vi "ZK流程写入.vi"(7 "是否启用通讯通知":bool, 8 "error in (no error)":errorcluster, 10 "流程":T1 {"进样流程"."进样流程-进样"."步骤二："."功能" items=["加标", "进样", "排液", "搅拌", "定量", "延时"]; "进样流程"."进样流程-进样"."步骤一："."功能" items=["加标", "进样", "排液", "搅拌", "定量", "延时"]; "进样流程"."进样流程-进样"."步骤四："."功能" items=["加标", "进样", "排液", "搅拌", "定量", "延时"]; "进样流程"."进样流程-进样"."步骤三："."功能" items=["加标", "进样", "排液", "搅拌", "定量", "延时"]; "进样流程"."进样流程-进样"."步骤六："."功能" items=["加标", "进样", "排液", "搅拌", "定量", "延时"]; "进样流程"."进样流程-进样"."步骤五："."功能" items=["加标", "进样", "排液", "搅拌", "定量", "延时"]; "进样流程"."进样流程-进样"."步骤八："."功能" items=["加标", "进样", "排液", "搅拌", "定量", "延时"]; "进样流程"."进样流程-进样"."步骤七："."功能" items=["加标", "进样", "排液", "搅拌", "定量", "延时"]; "进样流程"."进样流程-进样"."步骤十："."功能" items=["加标", "进样", "排液", "搅拌", "定量", "延时"]; "进样流程"."进样流程-进样"."步骤九："."功能" items=["加标", "进样", "排液", "搅拌", "定量", "延时"]; "进样流程"."进样流程-润洗"."步骤二："."功能" items=["加标", "进样", "排液", "搅拌", "定量", "延时"]; "进样流程"."进样流程-润洗"."步骤一："."功能" items=["加标", "进样", "排液", "搅拌", "定量", "延时"]; "进样流程"."进样流程-润洗"."步骤四："."功能" items=["加标", "进样", "排液", "搅拌", "定量", "延时"]; "进样流程"."进样流程-润洗"."步骤三："."功能" items=["加标", "进样", "排液", "搅拌", "定量", "延时"]; "进样流程"."进样流程-润洗"."步骤六："."功能" items=["加标", "进样", "排液", "搅拌", "定量", "延时"]; "进样流程"."进样流程-润洗"."步骤五："."功能" items=["加标", "进样", "排液", "搅拌", "定量", "延时"]; "进样流程"."进样流程-润洗"."步骤八："."功能" items=["加标", "进样", "排液", "搅拌", "定量", "延时"]; "进样流程"."进样流程-润洗"."步骤七："."功能" items=["加标", "进样", "排液", "搅拌", "定量", "延时"]; "进样流程"."进样流程-润洗"."步骤十："."功能" items=["加标", "进样", "排液", "搅拌", "定量", "延时"]; "进样流程"."进样流程-润洗"."步骤九："."功能" items=["加标", "进样", "排液", "搅拌", "定量", "延时"]; "排液流程"."步骤二："."功能" items=["加标", "进样", "排液", "搅拌", "定量", "延时"]; "排液流程"."步骤一："."功能" items=["加标", "进样", "排液", "搅拌", "定量", "延时"]; "排液流程"."步骤四："."功能" items=["加标", "进样", "排液", "搅拌", "定量", "延时"]; "排液流程"."步骤三："."功能" items=["加标", "进样", "排液", "搅拌", "定量", "延时"]; "排液流程"."步骤六："."功能" items=["加标", "进样", "排液", "搅拌", "定量", "延时"]; "排液流程"."步骤五："."功能" items=["加标", "进样", "排液", "搅拌", "定量", "延时"]; "排液流程"."步骤八："."功能" items=["加标", "进样", "排液", "搅拌", "定量", "延时"]; "排液流程"."步骤七："."功能" items=["加标", "进样", "排液", "搅拌", "定量", "延时"]; "排液流程"."步骤十："."功能" items=["加标", "进样", "排液", "搅拌", "定量", "延时"]; "排液流程"."步骤九："."功能" items=["加标", "进样", "排液", "搅拌", "定量", "延时"]; "加标流程"."加标流程-加标"."步骤二："."功能" items=["加标", "进样", "排液", "搅拌", "定量", "延时"]; "加标流程"."加标流程-加标"."步骤一："."功能" items=["加标", "进样", "排液", "搅拌", "定量", "延时"]; "加标流程"."加标流程-加标"."步骤四："."功能" items=["加标", "进样", "排液", "搅拌", "定量", "延时"]; "加标流程"."加标流程-加标"."步骤三："."功能" items=["加标", "进样", "排液", "搅拌", "定量", "延时"]; "加标流程"."加标流程-加标"."步骤六："."功能" items=["加标", "进样", "排液", "搅拌", "定量", "延时"]; "加标流程"."加标流程-加标"."步骤五："."功能" items=["加标", "进样", "排液", "搅拌", "定量", "延时"]; "加标流程"."加标流程-加标"."步骤八："."功能" items=["加标", "进样", "排液", "搅拌", "定量", "延时"]; "加标流程"."加标流程-加标"."步骤七："."功能" items=["加标", "进样", "排液", "搅拌", "定量", "延时"]; "加标流程"."加标流程-加标"."步骤十："."功能" items=["加标", "进样", "排液", "搅拌", "定量", "延时"]; "加标流程"."加标流程-加标"."步骤九："."功能" items=["加标", "进样", "排液", "搅拌", "定量", "延时"]; "加标流程"."加标流程-定量"."步骤二："."功能" items=["加标", "进样", "排液", "搅拌", "定量", "延时"]; "加标流程"."加标流程-定量"."步骤一："."功能" items=["加标", "进样", "排液", "搅拌", "定量", "延时"]; "加标流程"."加标流程-定量"."步骤四："."功能" items=["加标", "进样", "排液", "搅拌", "定量", "延时"]; "加标流程"."加标流程-定量"."步骤三："."功能" items=["加标", "进样", "排液", "搅拌", "定量", "延时"]; "加标流程"."加标流程-定量"."步骤六："."功能" items=["加标", "进样", "排液", "搅拌", "定量", "延时"]; "加标流程"."加标流程-定量"."步骤五："."功能" items=["加标", "进样", "排液", "搅拌", "定量", "延时"]; "加标流程"."加标流程-定量"."步骤八："."功能" items=["加标", "进样", "排液", "搅拌", "定量", "延时"]; "加标流程"."加标流程-定量"."步骤七："."功能" items=["加标", "进样", "排液", "搅拌", "定量", "延时"]; "加标流程"."加标流程-定量"."步骤十："."功能" items=["加标", "进样", "排液", "搅拌", "定量", "延时"]; "加标流程"."加标流程-定量"."步骤九："."功能" items=["加标", "进样", "排液", "搅拌", "定量", "延时"]; "加标流程"."加标流程-进样"."步骤二："."功能" items=["加标", "进样", "排液", "搅拌", "定量", "延时"]; "加标流程"."加标流程-进样"."步骤一："."功能" items=["加标", "进样", "排液", "搅拌", "定量", "延时"]; "加标流程"."加标流程-进样"."步骤四："."功能" items=["加标", "进样", "排液", "搅拌", "定量", "延时"]; "加标流程"."加标流程-进样"."步骤三："."功能" items=["加标", "进样", "排液", "搅拌", "定量", "延时"]; "加标流程"."加标流程-进样"."步骤六："."功能" items=["加标", "进样", "排液", "搅拌", "定量", "延时"]; "加标流程"."加标流程-进样"."步骤五："."功能" items=["加标", "进样", "排液", "搅拌", "定量", "延时"]; "加标流程"."加标流程-进样"."步骤八："."功能" items=["加标", "进样", "排液", "搅拌", "定量", "延时"]; "加标流程"."加标流程-进样"."步骤七："."功能" items=["加标", "进样", "排液", "搅拌", "定量", "延时"]; "加标流程"."加标流程-进样"."步骤十："."功能" items=["加标", "进样", "排液", "搅拌", "定量", "延时"]; "加标流程"."加标流程-进样"."步骤九："."功能" items=["加标", "进样", "排液", "搅拌", "定量", "延时"]; "加标流程"."加标流程-润洗"."步骤二："."功能" items=["加标", "进样", "排液", "搅拌", "定量", "延时"]; "加标流程"."加标流程-润洗"."步骤一："."功能" items=["加标", "进样", "排液", "搅拌", "定量", "延时"]; "加标流程"."加标流程-润洗"."步骤四："."功能" items=["加标", "进样", "排液", "搅拌", "定量", "延时"]; "加标流程"."加标流程-润洗"."步骤三："."功能" items=["加标", "进样", "排液", "搅拌", "定量", "延时"]; "加标流程"."加标流程-润洗"."步骤六："."功能" items=["加标", "进样", "排液", "搅拌", "定量", "延时"]; "加标流程"."加标流程-润洗"."步骤五："."功能" items=["加标", "进样", "排液", "搅拌", "定量", "延时"]; "加标流程"."加标流程-润洗"."步骤八："."功能" items=["加标", "进样", "排液", "搅拌", "定量", "延时"]; "加标流程"."加标流程-润洗"."步骤七："."功能" items=["加标", "进样", "排液", "搅拌", "定量", "延时"]; "加标流程"."加标流程-润洗"."步骤十："."功能" items=["加标", "进样", "排液", "搅拌", "定量", "延时"]; "加标流程"."加标流程-润洗"."步骤九："."功能" items=["加标", "进样", "排液", "搅拌", "定量", "延时"]; "加标润洗流程"."步骤二："."功能" items=["加标", "进样", "排液", "搅拌", "定量", "延时"]; "加标润洗流程"."步骤一："."功能" items=["加标", "进样", "排液", "搅拌", "定量", "延时"]; "加标润洗流程"."步骤四："."功能" items=["加标", "进样", "排液", "搅拌", "定量", "延时"]; "加标润洗流程"."步骤三："."功能" items=["加标", "进样", "排液", "搅拌", "定量", "延时"]; "加标润洗流程"."步骤六："."功能" items=["加标", "进样", "排液", "搅拌", "定量", "延时"]; "加标润洗流程"."步骤五："."功能" items=["加标", "进样", "排液", "搅拌", "定量", "延时"]; "加标润洗流程"."步骤八："."功能" items=["加标", "进样", "排液", "搅拌", "定量", "延时"]; "加标润洗流程"."步骤七："."功能" items=["加标", "进样", "排液", "搅拌", "定量", "延时"]; "加标润洗流程"."步骤十："."功能" items=["加标", "进样", "排液", "搅拌", "定量", "延时"]; "加标润洗流程"."步骤九："."功能" items=["加标", "进样", "排液", "搅拌", "定量", "延时"]; "水样润洗流程"."步骤二："."功能" items=["加标", "进样", "排液", "搅拌", "定量", "延时"]; "水样润洗流程"."步骤一："."功能" items=["加标", "进样", "排液", "搅拌", "定量", "延时"]; "水样润洗流程"."步骤四："."功能" items=["加标", "进样", "排液", "搅拌", "定量", "延时"]; "水样润洗流程"."步骤三："."功能" items=["加标", "进样", "排液", "搅拌", "定量", "延时"]; "水样润洗流程"."步骤六："."功能" items=["加标", "进样", "排液", "搅拌", "定量", "延时"]; "水样润洗流程"."步骤五："."功能" items=["加标", "进样", "排液", "搅拌", "定量", "延时"]; "水样润洗流程"."步骤八："."功能" items=["加标", "进样", "排液", "搅拌", "定量", "延时"]; "水样润洗流程"."步骤七："."功能" items=["加标", "进样", "排液", "搅拌", "定量", "延时"]; "水样润洗流程"."步骤十："."功能" items=["加标", "进样", "排液", "搅拌", "定量", "延时"]; "水样润洗流程"."步骤九："."功能" items=["加标", "进样", "排液", "搅拌", "定量", "延时"]}, 11 "Slave ID":T2) -> (0 "error out":errorcluster)   [LabVIEW 2016, in "质控单元V4.lvlib"]
uses:
  <vilib>/Plasmionique/MB Master/MB_Master/MB_Master.lvclass
  <vilib>/Plasmionique/MB Master/MB Master.lvlib
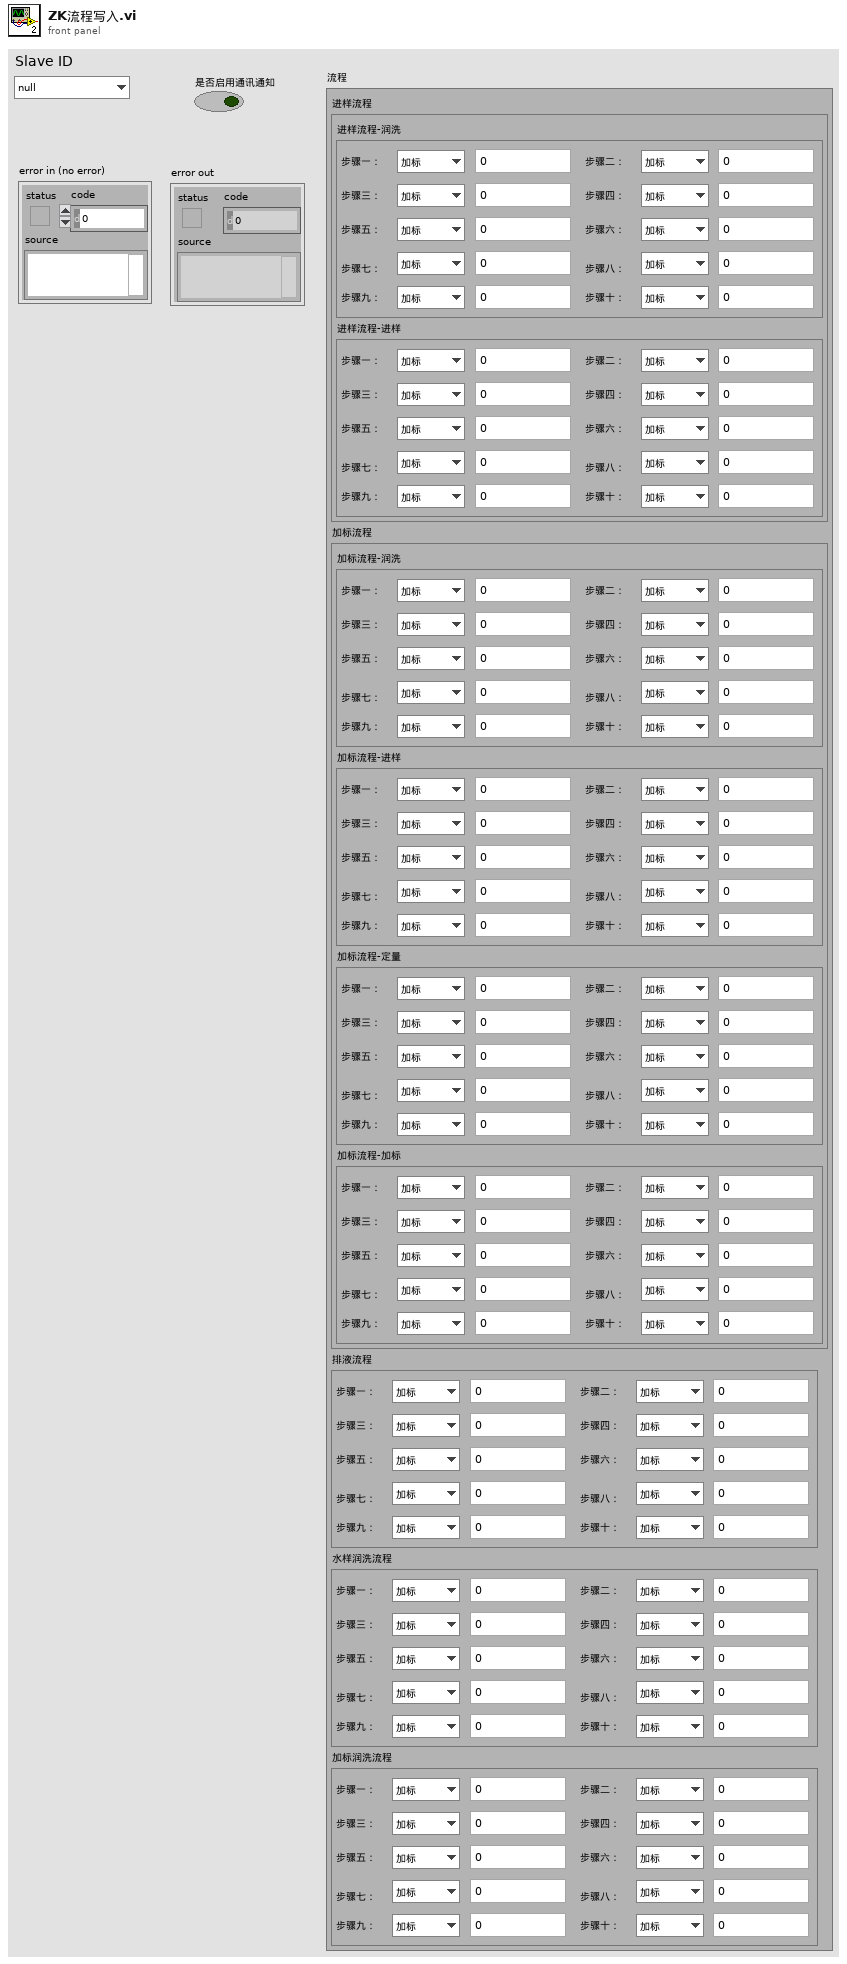
[diagram p1: front panel]
types:
  T1 = cluster{"进样流程":cluster{"进样流程-润洗":cluster{"步骤一：":cluster{"功能":u16, "值":sgl}, "步骤二：":cluster{"功能":u16, "值":sgl}, "步骤三：":cluster{"功能":u16, "值":sgl}, "步骤四：":cluster{"功能":u16, "值":sgl}, "步骤五：":cluster{"功能":u16, "值":sgl}, "步骤六：":cluster{"功能":u16, "值":sgl}, "步骤七：":cluster{"功能":u16, "值":sgl}, "步骤八：":cluster{"功能":u16, "值":sgl}, "步骤九：":cluster{"功能":u16, "值":sgl}, "步骤十：":cluster{"功能":u16, "值":sgl}}, "进样流程-进样":cluster{"步骤一：":cluster{"功能":u16, "值":sgl}, "步骤二：":cluster{"功能":u16, "值":sgl}, "步骤三：":cluster{"功能":u16, "值":sgl}, "步骤四：":cluster{"功能":u16, "值":sgl}, "步骤五：":cluster{"功能":u16, "值":sgl}, "步骤六：":cluster{"功能":u16, "值":sgl}, "步骤七：":cluster{"功能":u16, "值":sgl}, "步骤八：":cluster{"功能":u16, "值":sgl}, "步骤九：":cluster{"功能":u16, "值":sgl}, "步骤十：":cluster{"功能":u16, "值":sgl}}}, "加标流程":cluster{"加标流程-润洗":cluster{"步骤一：":cluster{"功能":u16, "值":sgl}, "步骤二：":cluster{"功能":u16, "值":sgl}, "步骤三：":cluster{"功能":u16, "值":sgl}, "步骤四：":cluster{"功能":u16, "值":sgl}, "步骤五：":cluster{"功能":u16, "值":sgl}, "步骤六：":cluster{"功能":u16, "值":sgl}, "步骤七：":cluster{"功能":u16, "值":sgl}, "步骤八：":cluster{"功能":u16, "值":sgl}, "步骤九：":cluster{"功能":u16, "值":sgl}, "步骤十：":cluster{"功能":u16, "值":sgl}}, "加标流程-进样":cluster{"步骤一：":cluster{"功能":u16, "值":sgl}, "步骤二：":cluster{"功能":u16, "值":sgl}, "步骤三：":cluster{"功能":u16, "值":sgl}, "步骤四：":cluster{"功能":u16, "值":sgl}, "步骤五：":cluster{"功能":u16, "值":sgl}, "步骤六：":cluster{"功能":u16, "值":sgl}, "步骤七：":cluster{"功能":u16, "值":sgl}, "步骤八：":cluster{"功能":u16, "值":sgl}, "步骤九：":cluster{"功能":u16, "值":sgl}, "步骤十：":cluster{"功能":u16, "值":sgl}}, "加标流程-定量":cluster{"步骤一：":cluster{"功能":u16, "值":sgl}, "步骤二：":cluster{"功能":u16, "值":sgl}, "步骤三：":cluster{"功能":u16, "值":sgl}, "步骤四：":cluster{"功能":u16, "值":sgl}, "步骤五：":cluster{"功能":u16, "值":sgl}, "步骤六：":cluster{"功能":u16, "值":sgl}, "步骤七：":cluster{"功能":u16, "值":sgl}, "步骤八：":cluster{"功能":u16, "值":sgl}, "步骤九：":cluster{"功能":u16, "值":sgl}, "步骤十：":cluster{"功能":u16, "值":sgl}}, "加标流程-加标":cluster{"步骤一：":cluster{"功能":u16, "值":sgl}, "步骤二：":cluster{"功能":u16, "值":sgl}, "步骤三：":cluster{"功能":u16, "值":sgl}, "步骤四：":cluster{"功能":u16, "值":sgl}, "步骤五：":cluster{"功能":u16, "值":sgl}, "步骤六：":cluster{"功能":u16, "值":sgl}, "步骤七：":cluster{"功能":u16, "值":sgl}, "步骤八：":cluster{"功能":u16, "值":sgl}, "步骤九：":cluster{"功能":u16, "值":sgl}, "步骤十：":cluster{"功能":u16, "值":sgl}}}, "排液流程":cluster{"步骤一：":cluster{"功能":u16, "值":sgl}, "步骤二：":cluster{"功能":u16, "值":sgl}, "步骤三：":cluster{"功能":u16, "值":sgl}, "步骤四：":cluster{"功能":u16, "值":sgl}, "步骤五：":cluster{"功能":u16, "值":sgl}, "步骤六：":cluster{"功能":u16, "值":sgl}, "步骤七：":cluster{"功能":u16, "值":sgl}, "步骤八：":cluster{"功能":u16, "值":sgl}, "步骤九：":cluster{"功能":u16, "值":sgl}, "步骤十：":cluster{"功能":u16, "值":sgl}}, "水样润洗流程":cluster{"步骤一：":cluster{"功能":u16, "值":sgl}, "步骤二：":cluster{"功能":u16, "值":sgl}, "步骤三：":cluster{"功能":u16, "值":sgl}, "步骤四：":cluster{"功能":u16, "值":sgl}, "步骤五：":cluster{"功能":u16, "值":sgl}, "步骤六：":cluster{"功能":u16, "值":sgl}, "步骤七：":cluster{"功能":u16, "值":sgl}, "步骤八：":cluster{"功能":u16, "值":sgl}, "步骤九：":cluster{"功能":u16, "值":sgl}, "步骤十：":cluster{"功能":u16, "值":sgl}}, "加标润洗流程":cluster{"步骤一：":cluster{"功能":u16, "值":sgl}, "步骤二：":cluster{"功能":u16, "值":sgl}, "步骤三：":cluster{"功能":u16, "值":sgl}, "步骤四：":cluster{"功能":u16, "值":sgl}, "步骤五：":cluster{"功能":u16, "值":sgl}, "步骤六：":cluster{"功能":u16, "值":sgl}, "步骤七：":cluster{"功能":u16, "值":sgl}, "步骤八：":cluster{"功能":u16, "值":sgl}, "步骤九：":cluster{"功能":u16, "值":sgl}, "步骤十：":cluster{"功能":u16, "值":sgl}}}
  T2 = typedef "质控单元V4.lvlib/质控slave id.ctl" = enum16{"null", "氨氮", "总磷", "总氮", "CODMn", "CODCr"}
  T3 = cluster{"步骤一：":cluster{"功能":u16, "值":sgl}, "步骤二：":cluster{"功能":u16, "值":sgl}, "步骤三：":cluster{"功能":u16, "值":sgl}, "步骤四：":cluster{"功能":u16, "值":sgl}, "步骤五：":cluster{"功能":u16, "值":sgl}, "步骤六：":cluster{"功能":u16, "值":sgl}, "步骤七：":cluster{"功能":u16, "值":sgl}, "步骤八：":cluster{"功能":u16, "值":sgl}, "步骤九：":cluster{"功能":u16, "值":sgl}, "步骤十：":cluster{"功能":u16, "值":sgl}}
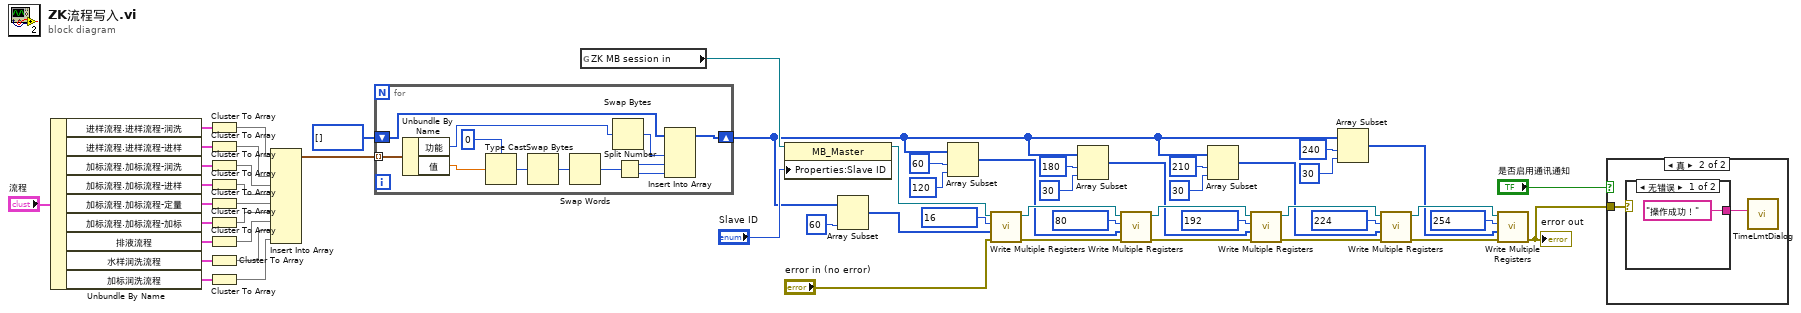
[diagram p0: block diagram]
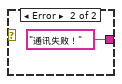
[diagram p3: hidden frame]
diagram:
  n1 = Unbundle By Name("流程") -> ("进样流程.进样流程-润洗"=w48:T3, "进样流程.进样流程-进样"=w46:T3, "加标流程.加标流程-润洗"=w45:T3, "加标流程.加标流程-进样"=w44:T3, "加标流程.加标流程-定量"=w43:T3, "加标流程.加标流程-加标"=w42:T3, "排液流程"=w41:T3, "水样润洗流程"=w40:T3, "加标润洗流程"=w39:T3)
  n2 = Cluster To Array(cluster=w48) -> (array=w38:cluster{"功能":u16, "值":sgl}[])
  n3 = Cluster To Array(cluster=w46) -> (array=w37:cluster{"功能":u16, "值":sgl}[])
  n4 = Cluster To Array(cluster=w45) -> (array=w36:cluster{"功能":u16, "值":sgl}[])
  n5 = Cluster To Array(cluster=w44) -> (array=w35:cluster{"功能":u16, "值":sgl}[])
  n6 = Cluster To Array(cluster=w43) -> (array=w34:cluster{"功能":u16, "值":sgl}[])
  n7 = Cluster To Array(cluster=w42) -> (array=w33:cluster{"功能":u16, "值":sgl}[])
  n8 = Cluster To Array(cluster=w41) -> (array=w32:cluster{"功能":u16, "值":sgl}[])
  n9 = Cluster To Array(cluster=w40) -> (array=w31:cluster{"功能":u16, "值":sgl}[])
  n10 = Cluster To Array(cluster=w39) -> (array=w30:cluster{"功能":u16, "值":sgl}[])
  n11 = Insert Into Array(array=w38, new element #1=w37, new element #2=w36, new element #3=w35, new element #4=w34, new element #5=w33, new element #6=w32, new element #7=w31, new element #8=w30) -> (w29:cluster{"功能":u16, "值":sgl}[])  [unwired: 1 in]
  n12 = for {
    tunnel: w29 -> [w67] mode=indexing
    shift-right: [w56] -> w19
    shift-left: u16[] [] ("values") -> [w61]
    n13 = Unbundle By Name(w67) -> ("功能"=w60:u16, "值"=w62:sgl)
    n14 = Type Cast(type=0, x=w62) -> (*(type *) &x=w64:i32)
    n15 = Swap Bytes(anything=w64) -> (byte swapped=w63:i32)
    n16 = Swap Words(1:w63) -> (0:w66:i32)
    n17 = Swap Bytes(anything=w60) -> (byte swapped=w59:u16)
    n18 = Split Number(x=w66) -> (hi(x)=w58:u16, lo(x)=w57:u16)
    n19 = Insert Into Array(array=w61, new element #1=w59, new element #2=w58, new element #3=w57) -> (w56:u16[])  [unwired: 1 in]
  }
  n20 = global read "ZK非断电保存全局变量.vi" "ZK MB session in"() -> (w54:refnum<class "MB_Master.lvclass">)
  n21 = property class="MB_Master"(reference=w54, "Properties:Slave ID"="Slave ID") -> (reference out=w52:refnum<class "MB_Master.lvclass">)  [unwired: 1 in, 1 out]
  n22 = Array Subset(array=w19, length=60 ("长度")) -> (w5:u16[])  [unwired: 1 in]
  n23 = Array Subset(array=w19, index=60 ("索引"), length=120 ("长度")) -> (w4:u16[])
  n24 = call <vilib>:"Write Multiple Registers.vi"("error in (no error)"="error in (no error)", "values"=w5, "starting address"=u16 16, "MB session in"=w52) -> ("error out"=w18:errorcluster, "MB session out"=w17:refnum<class "MB_Master.lvclass">)  [unwired: 6 in]
  n25 = Array Subset(array=w19, index=180 ("索引"), length=30 ("长度")) -> (w3:u16[])
  n26 = call <vilib>:"Write Multiple Registers.vi"("error in (no error)"=w18, "values"=w4, "starting address"=u16 80, "MB session in"=w17) -> ("error out"=w16:errorcluster, "MB session out"=w15:refnum<class "MB_Master.lvclass">)  [unwired: 6 in]
  n27 = Array Subset(array=w19, index=210 ("索引"), length=30 ("长度")) -> (w2:u16[])
  n28 = call <vilib>:"Write Multiple Registers.vi"("error in (no error)"=w16, "values"=w3, "starting address"=u16 192, "MB session in"=w15) -> ("error out"=w14:errorcluster, "MB session out"=w13:refnum<class "MB_Master.lvclass">)  [unwired: 6 in]
  n29 = Array Subset(array=w19, index=240 ("索引"), length=30 ("长度")) -> (w1:u16[])
  n30 = call <vilib>:"Write Multiple Registers.vi"("error in (no error)"=w14, "values"=w2, "starting address"=u16 224, "MB session in"=w13) -> ("error out"=w12:errorcluster, "MB session out"=w11:refnum<class "MB_Master.lvclass">)  [unwired: 6 in]
  n31 = call <vilib>:"Write Multiple Registers.vi"("error in (no error)"=w12, "values"=w1, "starting address"=u16 254, "MB session in"=w11) -> ("error out"=w10:errorcluster)  [unwired: 6 in, 1 out]
  "error out" <- w10
  n32 = case shown="真" "是否启用通讯通知" {
    tunnel: w10 -> [_ w69]
    frame False {
    }
    frame True {
      n33 = case shown="无错误" w69 {
        tunnel: ["操作成功！" "通讯失败！"] -> w68
        frame No Error {
        }
        frame Error {
        }
      }
      n34 = call "TimeLmtDialog.vi"("Infoin"=w68) -> ()  [unwired: 11 in]
    }
  }
